vi "TcpErrorHandler.vi"(8 "error in (no error)":errorcluster, 9 "consequtive error count in":i32, 11 "Qbus in":refnum<class "Qbus.lvclass">) -> (0 "error out":errorcluster, 1 "consequtive error count out":i32, 3 "Qbus out":refnum<class "Qbus.lvclass">)   [LabVIEW 2017, in "ServerComm.lvlib"]
uses:
  <vilib>/addons/InsightCM/Devices/Shared/Common/ServerComm/ServerComm.lvlib
  <vilib>/addons/Qbus/Qbus.lvclass
  <vilib>/addons/TraceLogger/TraceLogger.lvlib
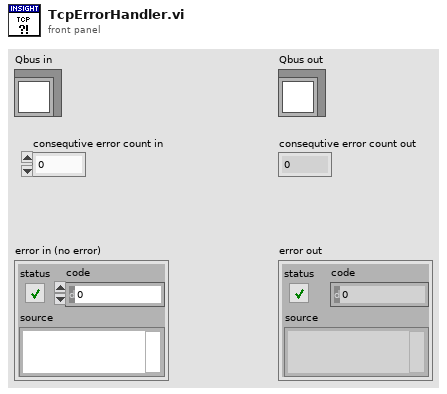
[diagram p1: front panel]
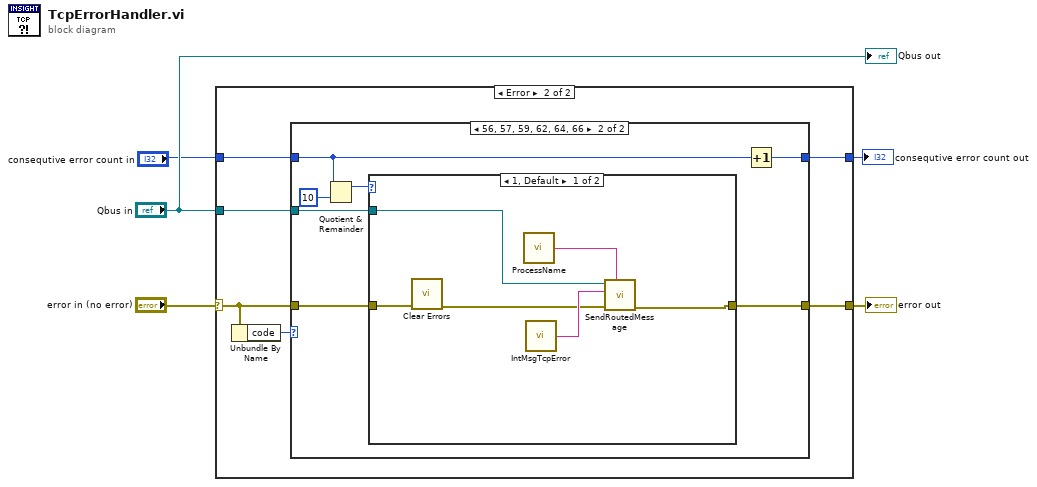
[diagram p0: block diagram]
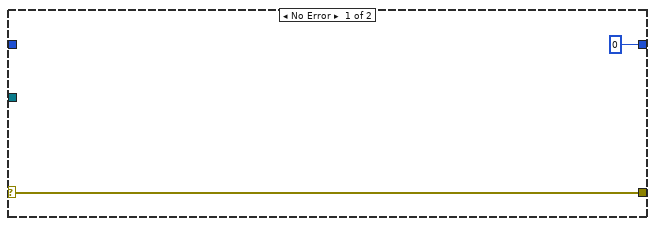
[diagram p2: hidden frame]
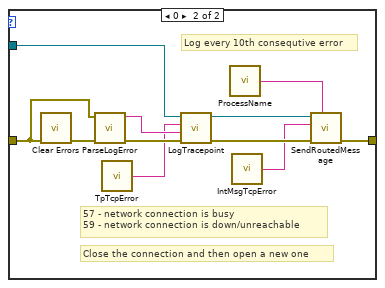
[diagram p4: hidden frame]
diagram:
  n1 = case shown="Error" "error in (no error)" {
    selector: "error in (no error)" -> [w7 w12]
    tunnel: [w7 w11] -> w4
    tunnel: "Qbus in" -> [_ w10]
    tunnel: [0 w9] -> w2
    tunnel: "consequtive error count in" -> [_ w8]
    frame No Error {
    }
    frame Error {
      n2 = Unbundle By Name(w12) -> ("code"=w13:i32)
      n3 = case shown="56, 57, 59, 62, 64, 66" w13 {
        tunnel: w12 -> [w15 w20]
        tunnel: [w15 w22] -> w11
        tunnel: w10 -> [_ w21]
        tunnel: [w14 w19] -> w9
        tunnel: w8 -> [w14 w18]
        frame Default {
        }
        frame 56, 57, 59, 62, 64, 66 {
          n4 = Quotient & Remainder(x=w18, y=10) -> (x-y*floor(x/y)=w16:i32)  [unwired: 1 out]
          n5 = case shown="1, Default" w16 {
            tunnel: [w25 w39] -> w22
            tunnel: w21 -> [w23 w36]
            tunnel: w20 -> [w28 w32]
            frame 1, Default {
              n6 = call <vilib>:"Clear Errors.vi"("error in (no error)"=w28) -> ("error out"=w26:errorcluster)  [unwired: 5 in, 1 out]
              n7 = call <vilib>:"ProcessName.vi"() -> ("process name"=w24:string)  [unwired: 5 in]
              n8 = call <vilib>:"IntMsgTcpError.vi"() -> ("message name"=w27:string)  [unwired: 5 in]
              n9 = call <vilib>:"SendRoutedMessage.vi"("listener process"=w24, "error in (no error)"=w26, "message name"=w27, "Qbus in"=w23) -> ("error in (no error)"=w25:errorcluster)  [unwired: 6 in, 1 out]
            }
            frame 0 {
              # "Log every 10th consequtive error"
              # "Close the connection and then open a new one"
              # "57 - network connection is busy\n59 - network connection is down/unreachable"
              n10 = call <vilib>:"Clear Errors.vi"("error in (no error)"=w32) -> ("error out"=w34:errorcluster)  [unwired: 5 in, 1 out]
              n11 = call <vilib>:"ParseLogError.vi"("error in (no error)"=w34, "message body"=w32) -> ("error out"=w33:errorcluster, "error string"=w31:string)  [unwired: 8 in]
              n12 = call <vilib>:"TpTcpError.vi"() -> ("tracepoint name"=w30:string)  [unwired: 5 in]
              n13 = call <vilib>:"LogTracepoint.vi"("error in (no error)"=w33, "log string"=w31, "tracepoint"=w30, "qbus in"=w36) -> ("error out"=w37:errorcluster, "qbus out"=w35:refnum<class "Qbus.lvclass">)  [unwired: 6 in]
              n14 = call <vilib>:"ProcessName.vi"() -> ("process name"=w38:string)  [unwired: 5 in]
              n15 = call <vilib>:"IntMsgTcpError.vi"() -> ("message name"=w29:string)  [unwired: 5 in]
              n16 = call <vilib>:"SendRoutedMessage.vi"("listener process"=w38, "error in (no error)"=w37, "message name"=w29, "Qbus in"=w35) -> ("error in (no error)"=w39:errorcluster)  [unwired: 6 in, 1 out]
            }
          }
          n17 = Increment(x=w18) -> (x+1=w19:i32)
        }
      }
    }
  }
  "error out" <- w4
  "consequtive error count out" <- w2
  "Qbus out" <- "Qbus in"
